vi "打开程序.vi"(8 "error in (no error)":errorcluster caption="错误输入（无错误）", 11 "程序 输入":refnum<class "程序.lvclass">) -> (0 "error out":errorcluster caption="错误输出", 3 "程序 输出":refnum<class "程序.lvclass">)   [LabVIEW 2020, in "程序.lvclass"]
uses:
  D:/SuperPython-master/ScintillaNET.dll
  ScintillaNET.dll
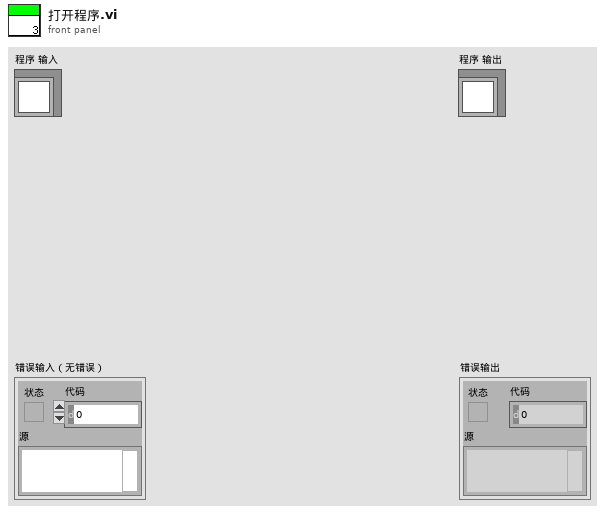
[diagram p1: front panel]
types:
  T1 = typedef "imagedata.ctl" = cluster{"image type":i32, "image depth":i32, "image":u8[], "mask":u8[], "colors":u32[], "Rectangle":cluster{"left":i16, "top":i16, "right":i16, "bottom":i16}}
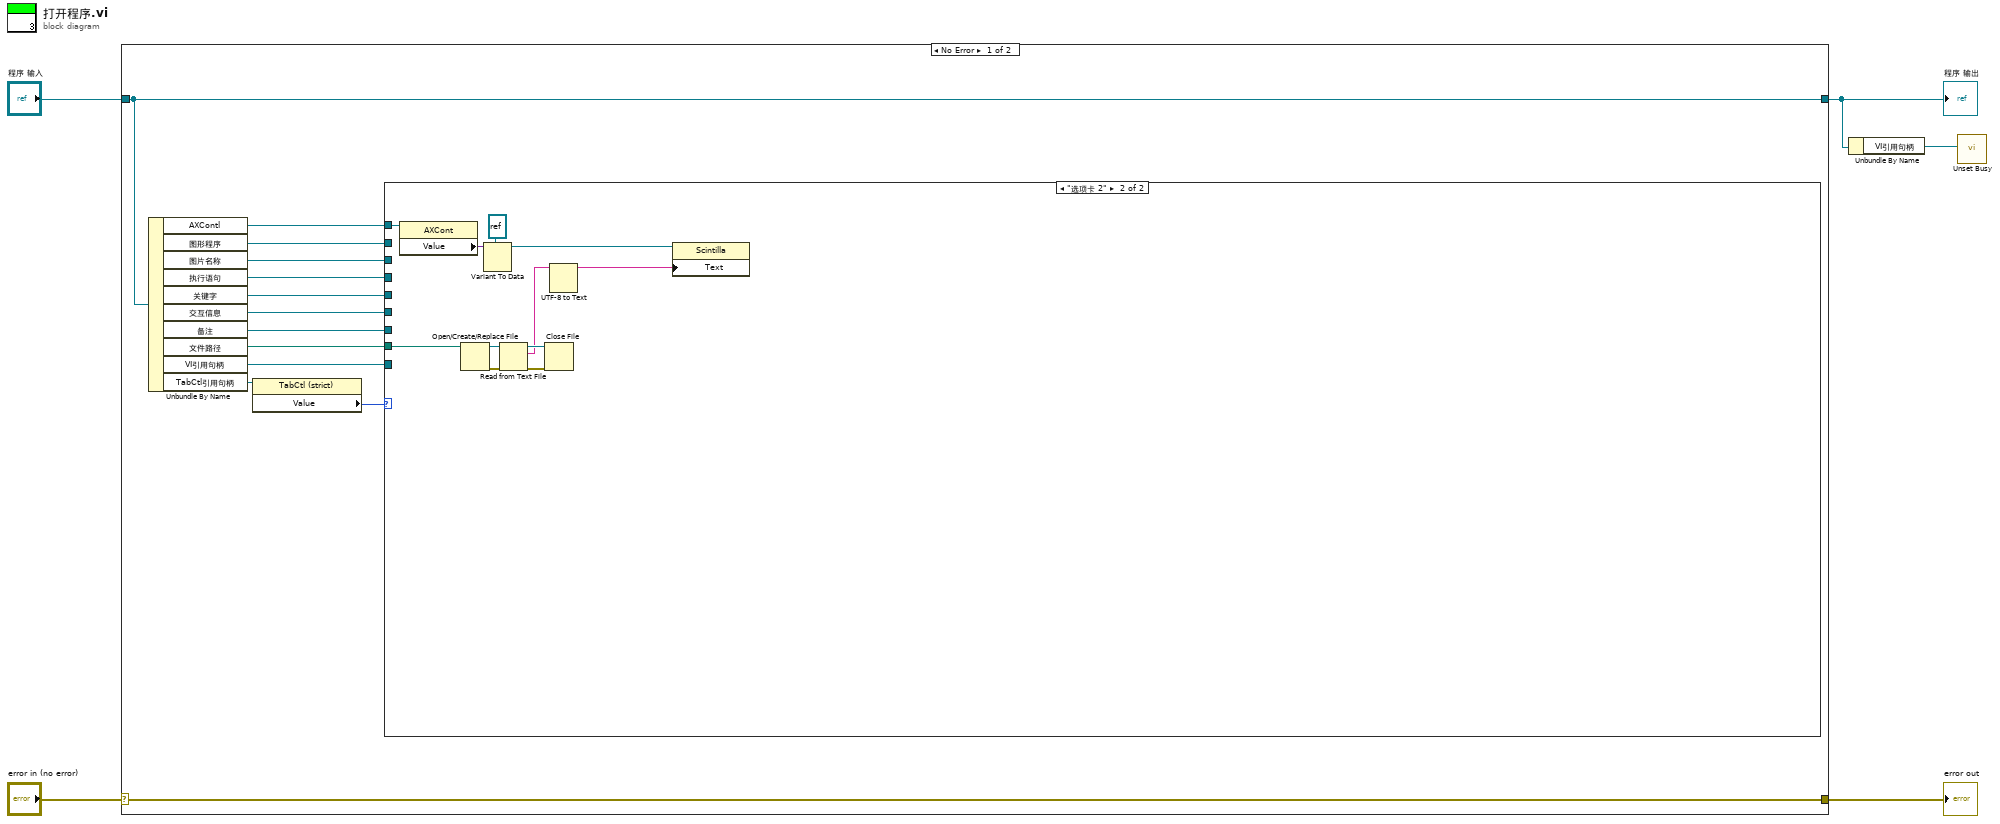
[diagram p0: block diagram]
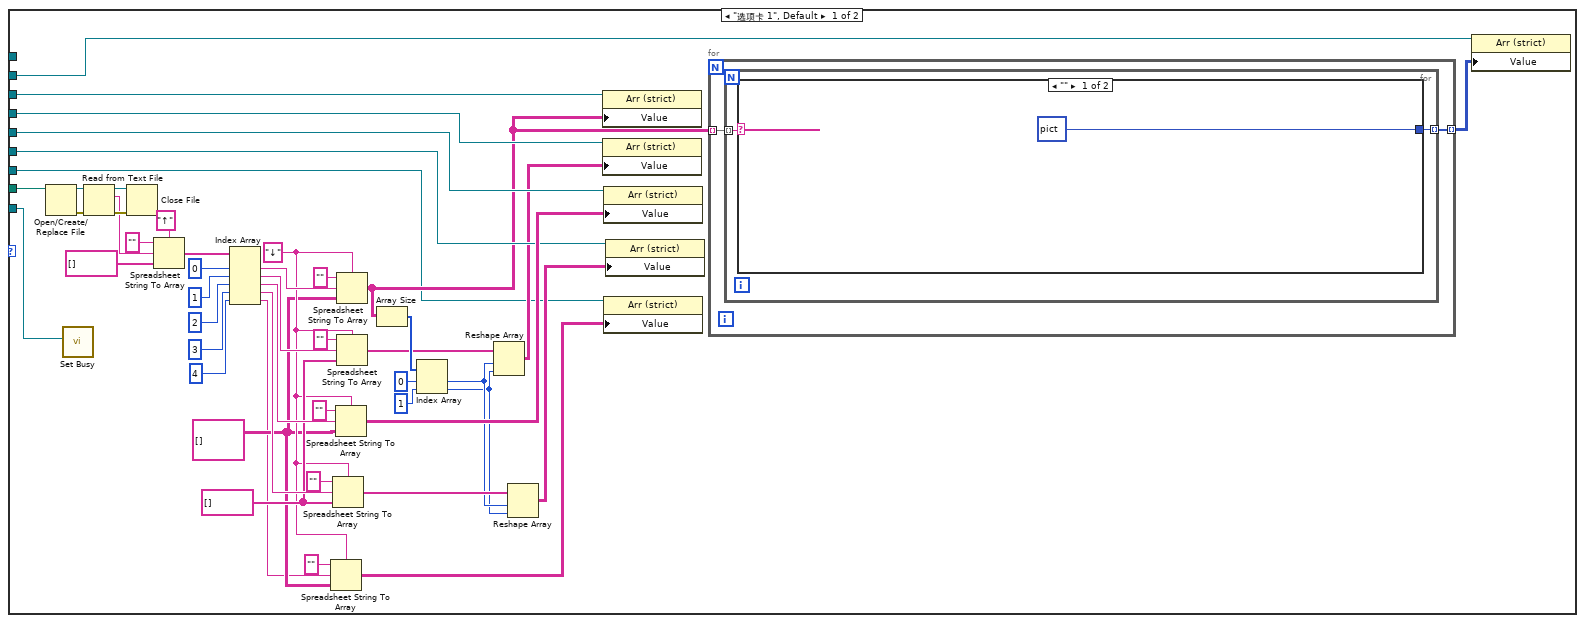
[diagram p2: hidden frame]
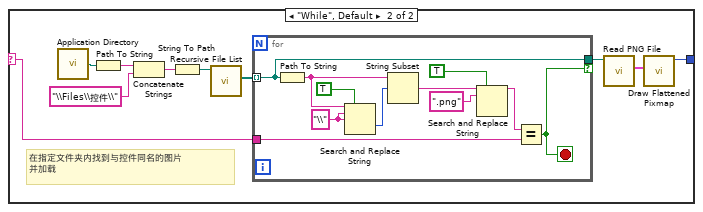
[diagram p3: hidden frame]
diagram:
  n1 = case shown="No Error" "error in (no error)" {
    selector: "error in (no error)" -> [w18 w105]
    tunnel: [w18 w105] -> w4
    tunnel: [w17 w104] -> w2
    tunnel: "程序 输入" -> [w17 w104]
    frame No Error {
      n2 = Unbundle By Name(w17) -> ("AXContl"=w6:refnum<vi>, "图形程序"=w12:refnum<vi>, "图片名称"=w15:refnum<vi>, "执行语句"=w14:refnum<vi>, "关键字"=w13:refnum<vi>, "交互信息"=w11:refnum<vi>, "备注"=w10:refnum<vi>, "文件路径"=w16:path, "VI引用句柄"=w9:refnum<vi>, "TabCtl引用句柄"=w8:refnum<vi>)
      n3 = property class="TabCtl (strict)"(reference=w8) -> ("Value"=w7:enum32{"选项卡 1", "选项卡 2"})  [unwired: 1 in, 2 out]
      n4 = case shown="\"选项卡 2\"" w7 {
        tunnel: w16 -> [w62 w101]
        tunnel: w15 -> [w53 _]
        tunnel: w14 -> [w46 _]
        tunnel: w13 -> [w45 _]
        tunnel: w12 -> [w44 _]
        tunnel: w11 -> [w38 _]
        tunnel: w10 -> [w21 _]
        tunnel: w9 -> [w19 _]
        tunnel: w6 -> [_ w98]
        frame "选项卡 1", Default {
          w24 = "↓" ("分隔符(Tab)")
          w32 = string[] []
          w23 = string[][] []
          n5 = Open/Create/Replace File(file path (use dialog)=w62) -> (refnum out=w66:refnum<file>, error out=w65:errorcluster)  [unwired: 5 in, 1 out]
          n6 = call <vilib>:"Set Busy.vi"("VI reference (current VI)"=w19) -> ()  [unwired: 9 in, 2 out]
          n7 = Read from Text File(file (use dialog)=w66, error in=w65) -> (refnum out=w64:refnum<file>, text=w58:string, error out=w63:errorcluster)  [unwired: 2 in, 1 out]
          n8 = Close File(refnum=w64, error in=w63) -> ()  [unwired: 2 out]
          n9 = Spreadsheet String To Array(delimiter (Tab)="↑" ("分隔符(Tab)"), format string="" ("格式字符串"), spreadsheet string=w58, array type (2D Dbl)=string[] []) -> (array=w57:string[])
          n10 = Index Array(array=w57, index #1=0 ("索引"), index #2=1 ("索引"), index #3=2 ("索引"), index #4=3 ("索引"), index #5=4 ("索引")) -> (element #1=w51:string, element #2=w50:string, element #3=w47:string, element #4=w39:string, element #5=w22:string)
          n11 = Spreadsheet String To Array(delimiter (Tab)=w24, format string="" ("格式字符串"), spreadsheet string=w22, array type (2D Dbl)=w23) -> (array=w20:string[][])
          n12 = Spreadsheet String To Array(delimiter (Tab)=w24, format string="" ("格式字符串"), spreadsheet string=w39, array type (2D Dbl)=w32) -> (array=w36:string[])
          n13 = Spreadsheet String To Array(delimiter (Tab)=w24, format string="" ("格式字符串"), spreadsheet string=w47, array type (2D Dbl)=w23) -> (array=w43:string[][])
          n14 = Spreadsheet String To Array(delimiter (Tab)=w24, format string="" ("格式字符串"), spreadsheet string=w51, array type (2D Dbl)=w23) -> (array=w37:string[][])
          n15 = Spreadsheet String To Array(delimiter (Tab)=w24, format string="" ("格式字符串"), spreadsheet string=w50, array type (2D Dbl)=w32) -> (array=w30:string[])
          n16 = Array Size(array=w37) -> (size(s)=w35:i32[])
          n17 = Index Array(array=w35, index #1=0 ("索引"), index #2=1 ("索引")) -> (element #1=w28:i32, element #2=w27:i32)
          n18 = Reshape Array(w30, w28, w27) -> (w29:string[][])
          n19 = Reshape Array(w36, w28, w27) -> (w31:string[][])
          n20 = property class="Arr (strict)"(reference=w53, "Value"=w37) -> ()  [unwired: 1 in, 2 out]
          n21 = property class="Arr (strict)"(reference=w46, "Value"=w29) -> ()  [unwired: 1 in, 2 out]
          n22 = property class="Arr (strict)"(reference=w45, "Value"=w43) -> ()  [unwired: 1 in, 2 out]
          n23 = property class="Arr (strict)"(reference=w21, "Value"=w20) -> ()  [unwired: 1 in, 2 out]
          n24 = property class="Arr (strict)"(reference=w38, "Value"=w31) -> ()  [unwired: 1 in, 2 out]
          n25 = for {
            tunnel: w37 -> [w68] mode=indexing
            tunnel: [w67] -> w42 mode=indexing
            n26 = for {
              tunnel: w68 -> [w70] mode=indexing
              tunnel: [w69] -> w67 mode=indexing
              n27 = case shown="\"\"" w70 {
                selector: w70 -> [_ w73]
                tunnel: [picture data[5B] ("二维图片") w80] -> w69
                frame "" {
                }
                frame "While", Default {
                  # "在指定文件夹内找到与控件同名的图片\n并加载"
                  n28 = call <vilib>:"Application Directory.vi"() -> ("Application Directory"=w74:path)
                  n29 = Path To String(path=w74) -> (string=w77:string)
                  n30 = Concatenate Strings(w77, "\\Files\\控件\\" ("名称或相对路径")) -> (w76:string)
                  n31 = String To Path(string=w76) -> (path=w78:path)
                  n32 = call <vilib>:"Recursive File List.vi"("Folder Path"=w78) -> ("All Files in Dir"=w79:path[])  [unwired: 6 in, 4 out]
                  n33 = for {
                    tunnel: w79 -> [w85] mode=indexing
                    tunnel: [w85] -> w72 if=w82
                    tunnel: w73 -> [w83]
                    stop <- w82 stop-if-true
                    w91 = "\\" ("搜索字符串")
                    n34 = Path To String(path=w85) -> (string=w90:string)
                    n35 = Search and Replace String(replace all?=TRUE ("替换全部？(F)"), input string=w90, search string=w91, replace string=w91) -> (offset past replacement=w89:i32)  [unwired: 4 in, 3 out]
                    n36 = String Subset(string=w90, offset (0)=w89) -> (substring=w87:string)  [unwired: 1 in]
                    n37 = Search and Replace String(replace all?=TRUE ("替换全部？(F)"), input string=w87, search string=".png" ("搜索字符串")) -> (result string=w84:string)  [unwired: 5 in, 3 out]
                    n38 = Equal?(x=w84, y=w83) -> (x = y?=w82:bool)
                  }
                  n39 = call <vilib>:"Read PNG File.vi"("path to PNG file"=w72) -> ("image data"=w81:T1)  [unwired: 8 in, 2 out]
                  n40 = call <vilib>:"Draw Flattened Pixmap.vi"("image data"=w81) -> ("new picture"=w80:picture)  [unwired: 8 in]
                }
              }
            }
          }
          n41 = property class="Arr (strict)"(reference=w44, "Value"=w42) -> ()  [unwired: 1 in, 2 out]
        }
        frame "选项卡 2" {
          n42 = property class="AXCont"(reference=w98) -> ("Value"=w95:variant)  [unwired: 1 in, 2 out]
          n43 = Open/Create/Replace File(file path (use dialog)=w101) -> (refnum out=w103:refnum<file>, error out=w100:errorcluster)  [unwired: 5 in, 1 out]
          n44 = Variant To Data(type=refnum<k24> refnum ("文本编辑"), Variant=w95) -> (data=w96:refnum<k24>)  [unwired: 1 in, 1 out]
          n45 = Read from Text File(file (use dialog)=w103, error in=w100) -> (refnum out=w102:refnum<file>, text=w94:string, error out=w99:errorcluster)  [unwired: 2 in, 1 out]
          n46 = Close File(refnum=w102, error in=w99) -> ()  [unwired: 2 out]
          n47 = UTF-8 to Text ("UTF-8至文本转换")(11:w94) -> (3:w93:string)  [unwired: 2 in, 1 out]
          n48 = property class="Scintilla"(reference=w96, "Text"=w93) -> ()  [unwired: 1 in, 2 out]
        }
      }
    }
    frame Error {
    }
  }
  "error out" <- w4
  "程序 输出" <- w2
  n49 = Unbundle By Name(w2) -> ("VI引用句柄"=w1:refnum<vi>)
  n50 = call <vilib>:"Unset Busy.vi"("VI reference (current VI)"=w1) -> ()  [unwired: 10 in, 1 out]
